vi "Configure Measurement Histogram (N Cycle Jitter).vi"(0 "VISA resource name":refnum<visa-resource-name>, 1 "Enable Measurement Histogram (Enable)":bool, 2 "Number Cycle (5)":u32, 3 "Start Cycle (1)":u32, 5 "Channel (1: Channel 1)":i32(ring) items=["Channel 1", "Channel 2", "Channel 3", "Channel 4", "Function 1", "Function 2", "Function 3", "Function 4", "Memory 1", "Memory 2", "Memory 3", "Memory 4"], 7 "Edge (0: Rising)":i32(ring) items=["Rising", "Falling"], 11 "error in (no error)":errorcluster) -> (4 "VISA resource name out":refnum<visa-resource-name>, 15 "error out":errorcluster)   [LabVIEW 2009, in "Agilent 8000 Series.lvlib"]
doc: "Configures the N C Jitter measurement and enables the Measurement Histogram Jitter analysis on it.\n\n<B>Note:</B>\nCalling this VI disables all previously enabled measurements and clears existing measurement results from display."
uses:
  Agilent 8000 Series.lvlib
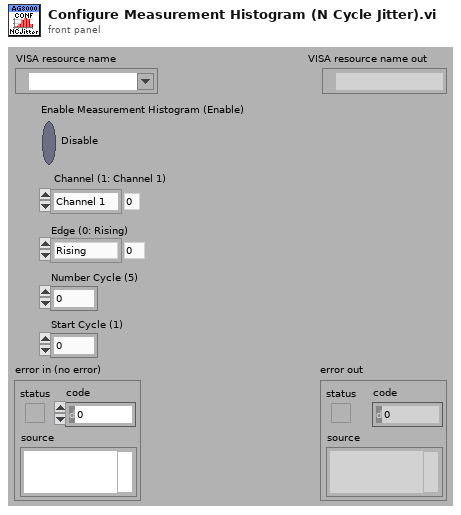
[diagram p1: front panel]
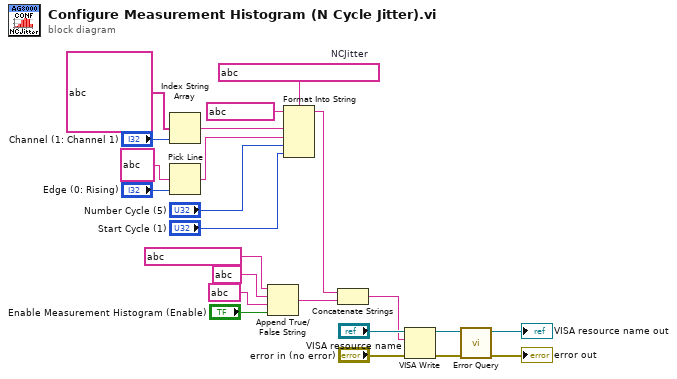
[diagram p0: block diagram]
diagram:
  w16 = string ?  # NCJitter
  n1 = Index String Array(1:"Channel (1: Channel 1)", 2:string[] ?) -> (0:w14:string)  [unwired: 1 in]
  n2 = Pick Line(multi-line string=string ?, line index="Edge (0: Rising)") -> (output string=w10:string)  [unwired: 1 in]
  n3 = Append True/False String(1:"Enable Measurement Histogram (Enable)", 2:string ? ("false string"), 3:string ? ("true string"), 4:string ? ("string (\"\")")) -> (0:w1:string)
  n4 = Format Into String(format string=w16, initial string=string ?, w14, w10, "Number Cycle (5)", "Start Cycle (1)") -> (resulting string=w2:string)  [unwired: 1 in, 1 out]
  n5 = Concatenate Strings(w2, w1) -> (w3:string)
  n6 = VISA Write(VISA resource name="VISA resource name", write buffer=w3, error in (no error)="error in (no error)") -> (VISA resource name out=w19:refnum<visa-resource-name>, error out=w18:errorcluster)  [unwired: 1 out]
  n7 = call "Error Query.vi"("error in (no error)"=w18, "VISA resource name"=w19) -> ("error out"=→"error out":errorcluster, "VISA resource name out"=→"VISA resource name out":refnum<visa-resource-name>)  [unwired: 6 in, 2 out]
